vi "[SubVI]Soft_Limit.vi"(5 "Motor Enable in":bool, 6 "Left Torque":dbl, 7 "Right Torque":dbl) -> (0 "PWM out":bool, 1 "ENA out":bool, 2 "L.SLimit":bool, 3 "R.SLimit":bool)   [LabVIEW 2019]
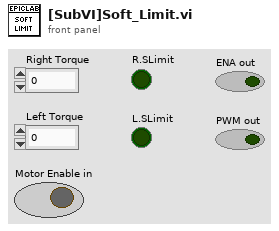
[diagram p1: front panel]
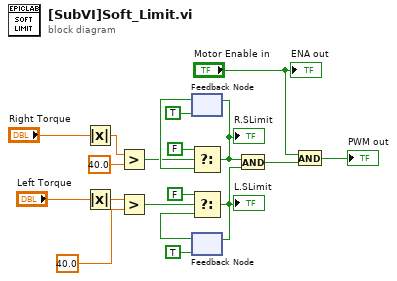
[diagram p0: block diagram]
diagram:
  n1 = Absolute Value(x="Right Torque") -> (abs(x)=w5:dbl)
  n2 = Absolute Value(x="Left Torque") -> (abs(x)=w2:dbl)
  n3 = Greater?(x=w5, y=40.0) -> (0:w6:bool)
  n4 = Greater?(x=w2, y=40.0) -> (0:w3:bool)
  n5 = feedback #1(TRUE) -> (w12:bool)
  n6 = Select(t=FALSE, s=w6, f=w12) -> (s? t:f=w11:bool)
  "R.SLimit" <- w11
  n7 = feedback-in #1(w11) -> ()
  n8 = feedback #2(TRUE) -> (w13:bool)
  n9 = Select(t=FALSE, s=w3, f=w13) -> (s? t:f=w14:bool)
  "L.SLimit" <- w14
  n10 = feedback-in #2(w14) -> ()
  n11 = And(x=w11, y=w14) -> (x .and. y?=w8:bool)
  n12 = And(x="Motor Enable in", y=w8) -> (x .and. y?=→"PWM out":bool)
  "ENA out" <- "Motor Enable in"
